vi "FGV-Counter.vi"(1 "Option":enum16{"Reset", "Get Current", "Count"}(ring)=enum."Get Current") -> (0 "output":i32)   [LabVIEW 2017]
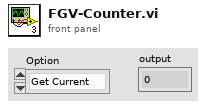
[diagram p1: front panel]
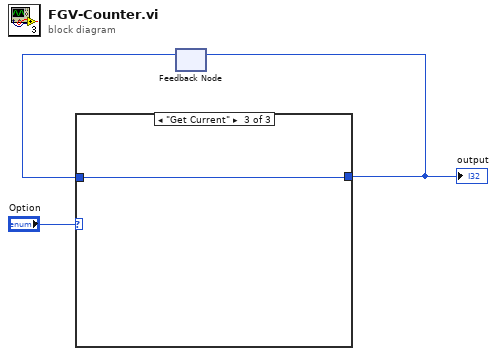
[diagram p0: block diagram]
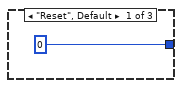
[diagram p2: hidden frame]
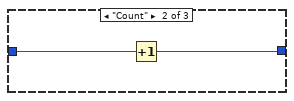
[diagram p3: hidden frame]
diagram:
  n1 = feedback #1() -> (w1:i32)  [unwired: 1 in]
  n2 = case shown="\"Get Current\"" "Option" {
    tunnel: [0 w5 w7] -> w2
    tunnel: w1 -> [_ w6 w7]
    frame "Reset", Default {
    }
    frame "Count" {
      n3 = Increment(x=w6) -> (x+1=w5:i32)
    }
    frame "Get Current" {
    }
  }
  "output" <- w2
  n4 = feedback-in #1(w2) -> ()
